vi "Test Acquisition API.vi"() -> ()   [LabVIEW 2019]
doc: "Acquisition API Tester.\n_____\nBased on DQMH Project Template 6.1.0.94."
uses:
  <vilib>/Utility/error.llb/DialogType.ctl
  Acquisition.lvlib
  Settings Editor/Settings Editor.lvlib
panel:
  in  "Command_GndImpedanceData":bool
  in  "Start EOC Acquiring":bool
  in  "Start CNV Acquiring":bool
  in  "IMP data updated":bool
  in  "Start GND Loop acquiring":bool
  in  "Stop IMP acquiring":bool
  in  "Start IMP Acquiring":bool
  in  "Soft Trigger":bool
  in  "Command_GoToIdle":bool
  in  "Command_ImpedanceData":bool
  in  "Command_LiveData":bool
  in  "Command_NoiseData":bool
  in  "Check WiFi AP":bool
  in  "Command_TestData":bool
  in  "Show Diagram on Init":bool
  in  "Settings":bool
  out "error out":errorcluster
  out "Calibrated?":bool
  in  "Calibrate":bool
  out "Waveform Chart":dbl(graph)
  out "Acquiring?":bool
  in  "Stop Acquiring":bool
  out "HW ID":string
  in  "Start Acquiring":bool
  in  "Show Block Diagram":bool
  in  "Stop Module":bool
  in  "Start Module":bool
  in  "Hide Module Panel":bool
  in  "Show Module Panel":bool
  out "Status":string
  out "Module Running?":bool
  # "This VI tests the API for the Module."
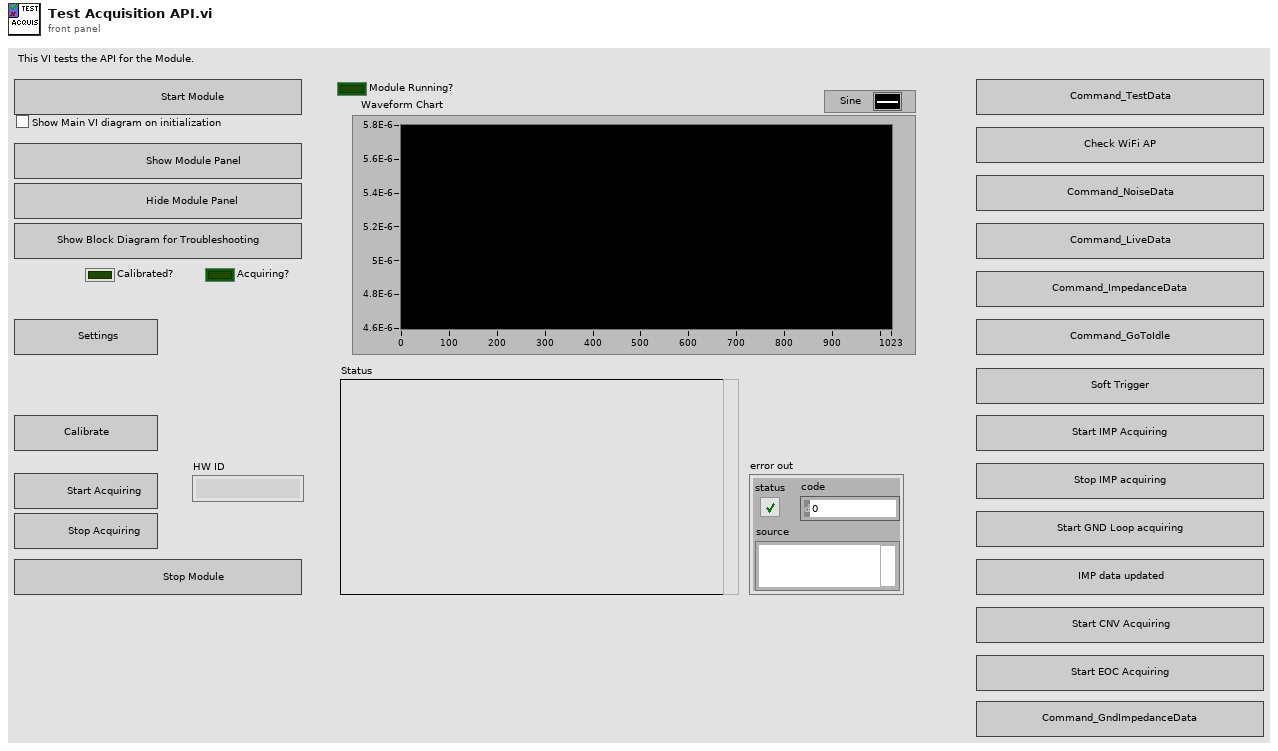
[diagram p1: front panel]
types:
  T1 = typedef "Acquisition.lvlib/Broadcast Events--cluster.ctl" = cluster{"Module Did Init":refnum<user-event>, "Status Updated":refnum<user-event>, "Error Reported":refnum<user-event>, "Module Did Stop":refnum<user-event>, "Update Module Execution Status":refnum<user-event>, "Acquisition Started":refnum<user-event>, "Acquisition Stopped":refnum<user-event>, "Data Updated":refnum<user-event>, "Device Calibrated":refnum<user-event>, "Impedance Data Updated":refnum<user-event>, "CNV Data Updated":refnum<user-event>, "EOC Data Updated":refnum<user-event>}
  T2 = typedef "DialogType.ctl" = u16
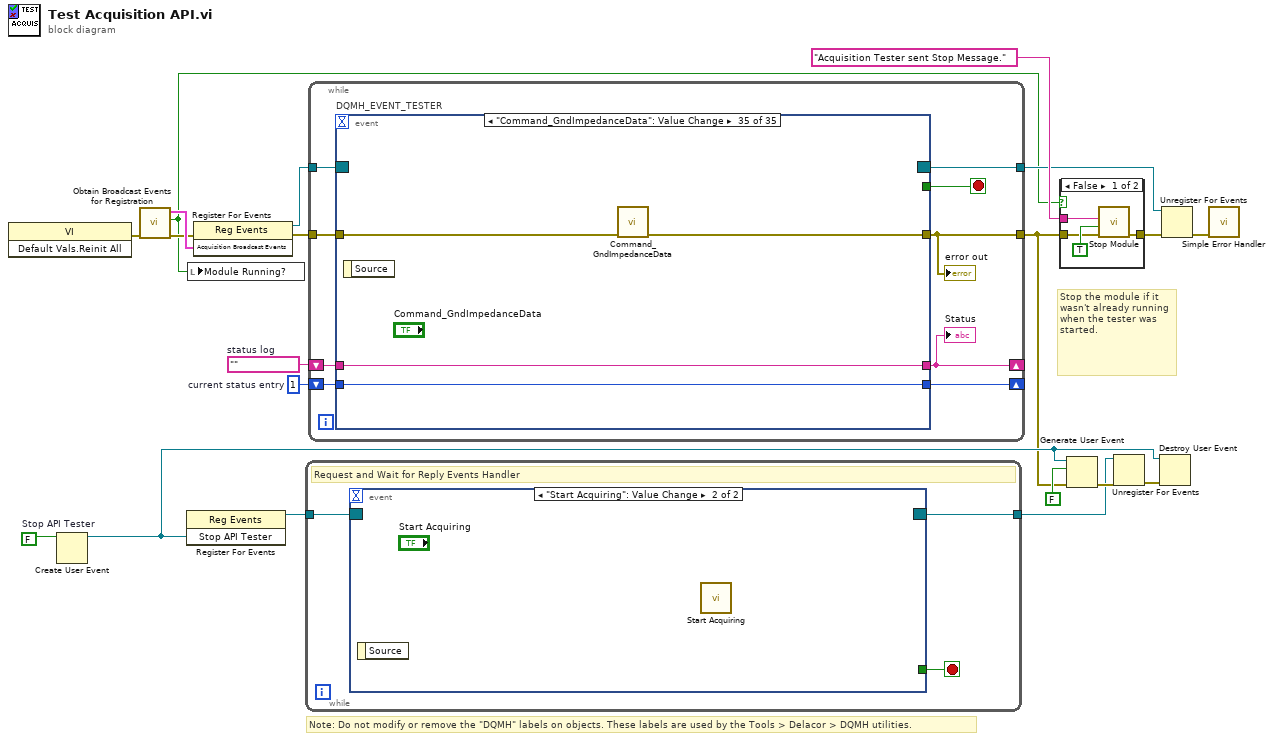
[diagram p0: block diagram]
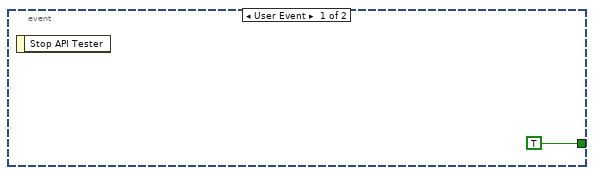
[diagram p2: hidden frame]
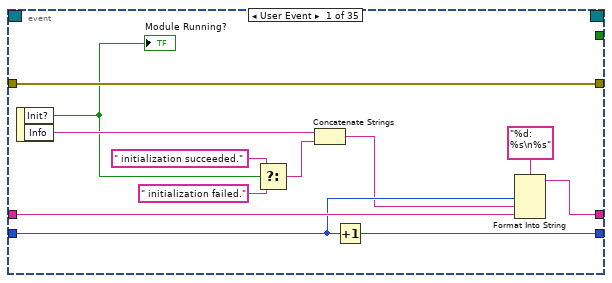
[diagram p3: hidden frame]
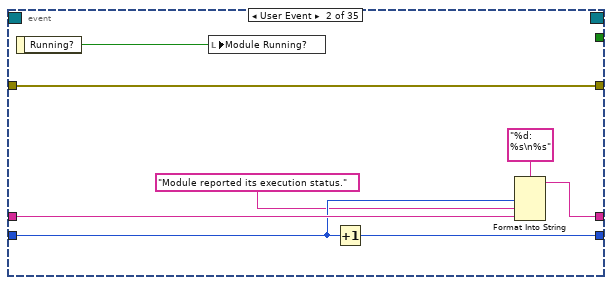
[diagram p4: hidden frame]
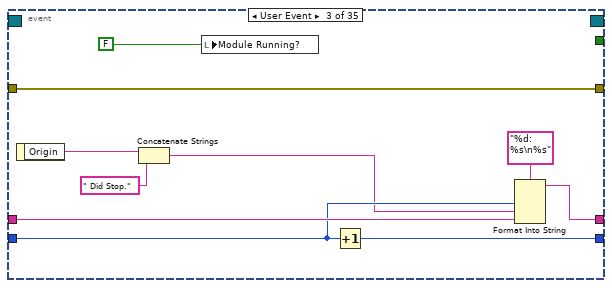
[diagram p5: hidden frame]
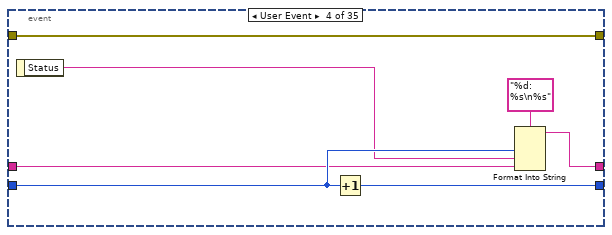
[diagram p6: hidden frame]
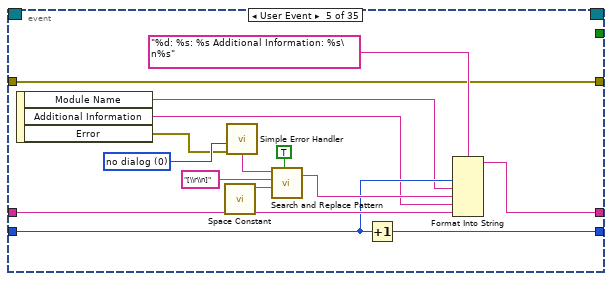
[diagram p7: hidden frame]
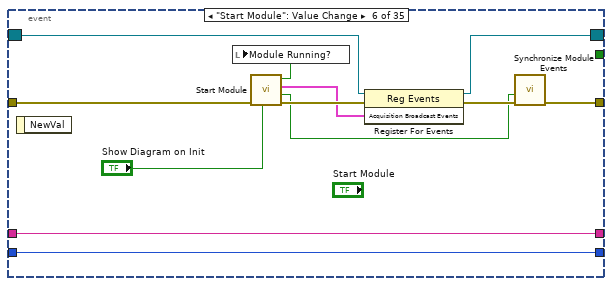
[diagram p8: hidden frame]
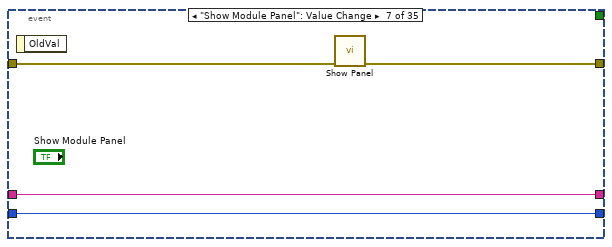
[diagram p9: hidden frame]
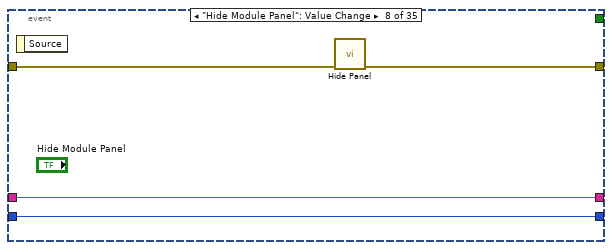
[diagram p10: hidden frame]
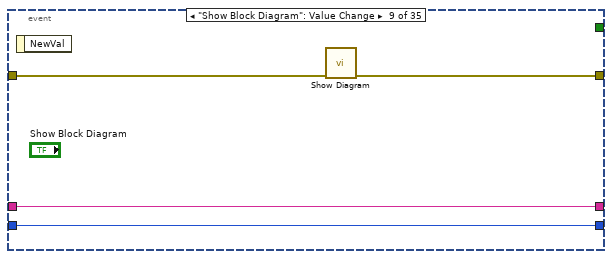
[diagram p11: hidden frame]
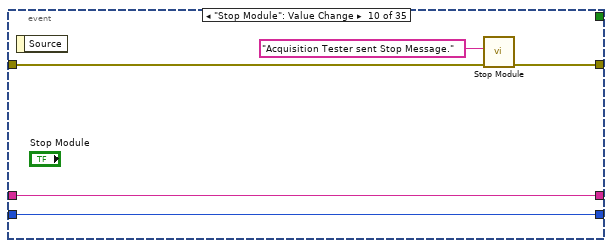
[diagram p12: hidden frame]
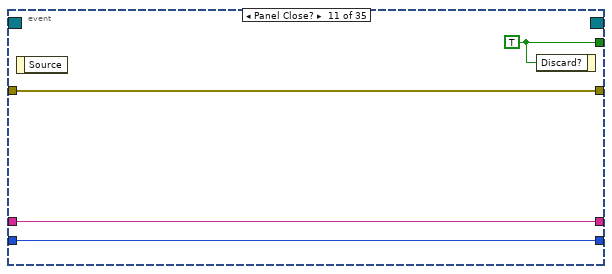
[diagram p13: hidden frame]
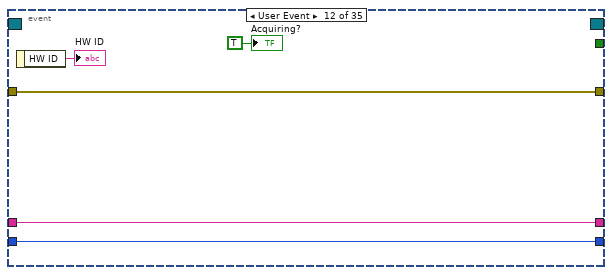
[diagram p14: hidden frame]
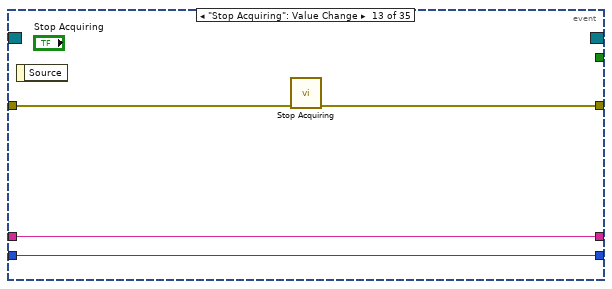
[diagram p15: hidden frame]
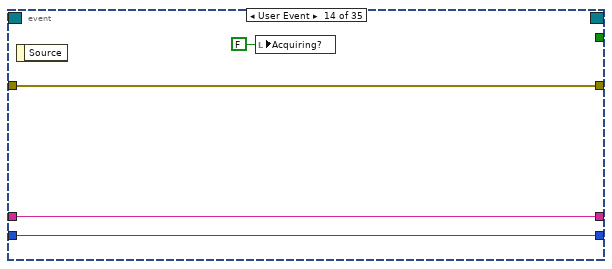
[diagram p16: hidden frame]
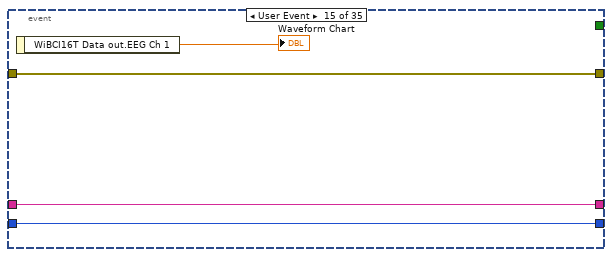
[diagram p17: hidden frame]
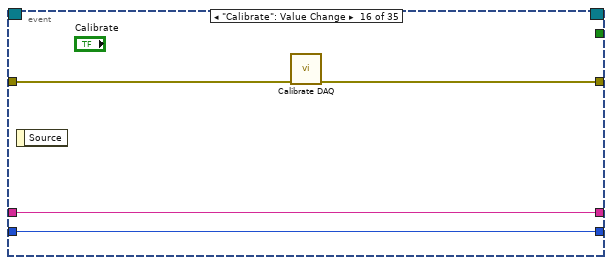
[diagram p18: hidden frame]
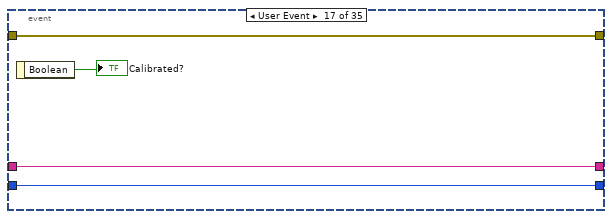
[diagram p19: hidden frame]
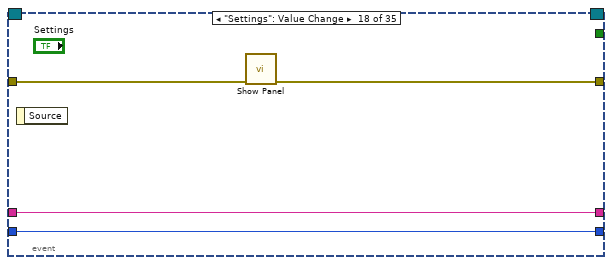
[diagram p20: hidden frame]
diagram:
  w10 = FALSE  # Stop API Tester
  w17 = 1  # current status entry
  w18 = ""  # status log
  # "Stop the module if it wasn't already running when the tester was started."
  # "Note: Do not modify or remove the \"DQMH\" labels on objects. These labels are used by the Tools > Delacor > DQMH utilities."
  n1 = invoke on="Invoke Node" class="VI" method="Default Vals.Reinit All"() -> (error out=w12:errorcluster)  [unwired: 3 in, 2 out]
  n2 = Create User Event(user event datatype=w10) -> (user event=w4:refnum<user-event>)  [unwired: 1 in, 1 out]
  n3 = call "Obtain Broadcast Events for Registration.vi"("error in"=w12) -> ("error out"=w11:errorcluster, "Already running?"=w3:bool, "Acquisition Broadcast Events"=w15:T1)  [unwired: 8 in]
  n4 = register-events(w4) -> (reference out=w9:refnum<event-registration>)  [unwired: 2 in, 1 out]
  n5 = local write "Module Running?"(w3) -> ()
  n6 = register-events(error in=w11, w15) -> (reference out=w14:refnum<event-registration>, error out=w16:errorcluster)  [unwired: 1 in]
  n7 = while {
    tunnel: w9 -> [w23]
    tunnel: [w21] -> w6
    stop <- w22 stop-if-true
    # "Request and Wait for Reply Events Handler"
    n8 = event shown="[1] \"Start Acquiring\": Value Change" {
      selector: w23 -> [_ _]
      dyn-events: [_ _] -> w21
      timeout: _ -> [_ _]
      tunnel: [TRUE _] -> w22
      event User Event {
        n9 = event-data() -> ()  [unwired: 1 in, 1 out]
      }
      event "Start Acquiring": Value Change {
        n10 = event-data() -> ()  [unwired: 1 in, 1 out]
        n11 = call "Start Acquiring.vi"() -> ()  [unwired: 9 in, 3 out]
      }
    }
  }
  n12 = while {
    tunnel: w14 -> [w33]
    tunnel: [w26] -> w2
    shift-right: [w29] -> _
    shift-left: w18 -> [w31]
    shift-right: [w30] -> _
    shift-left: w17 -> [w32]
    tunnel: w16 -> [w28]
    tunnel: [w27] -> w13
    stop <- w25 stop-if-true
    n13 = event "DQMH_EVENT_TESTER" shown="[34] \"Command_GndImpedanceData\": Value Change" {
      selector: w33 -> [_ _ _ _ _ w91 _ _ _ _ _ _ _ _ _ _ _ _ _ _ _ _ _ _ _ _ _ _ _ _ _ _ _ _ _]
      dyn-events: [_ _ _ _ _ w90 _ _ _ _ _ _ _ _ _ _ _ _ _ _ _ _ _ _ _ _ _ _ _ _ _ _ _ _ _] -> w27
      timeout: _ -> [_ _ _ _ _ _ _ _ _ _ _ _ _ _ _ _ _ _ _ _ _ _ _ _ _ _ _ _ _ _ _ _ _ _ _]
      tunnel: [_ _ _ _ _ _ _ _ _ _ w118 _ _ _ _ _ _ _ _ _ _ _ _ _ _ _ _ _ _ _ _ _ _ _ _] -> w25
      tunnel: [w45 w47 w54 w64 w74 w89 w101 w105 w106 w112 w115 w123 w124 w131 w135 w136 w143 w144 w148 w152 w156 w160 w164 w168 w173 w177 w181 w185 w189 w199 w208 w209 w213 w225 w226] -> w26
      tunnel: w32 -> [w42 w51 w61 w67 w77 w94 w99 w103 w107 w113 w116 w121 w125 w129 w133 w137 w141 w146 w149 w153 w157 w161 w165 w169 w174 w178 w182 w186 w190 w196 w205 w210 w214 w222 w227]
      tunnel: w31 -> [w43 w52 w62 w66 w78 w95 w100 w104 w108 w114 w117 w122 w126 w130 w134 w138 w142 w147 w150 w154 w158 w162 w166 w170 w175 w179 w183 w187 w191 w198 w207 w211 w215 w224 w228]
      tunnel: [w40 w49 w59 w68 w75 w95 w100 w104 w108 w114 w117 w122 w126 w130 w134 w138 w142 w147 w150 w154 w158 w162 w166 w170 w175 w179 w183 w187 w191 w197 w206 w211 w215 w223 w228] -> w29
      tunnel: [w41 w50 w60 w70 w76 w94 w99 w103 w107 w113 w116 w121 w125 w129 w133 w137 w141 w146 w149 w153 w157 w161 w165 w169 w174 w178 w182 w186 w190 w195 w204 w210 w214 w221 w227] -> w30
      tunnel: w28 -> [w45 w47 w54 w64 w74 w88 w98 w102 w109 w110 w115 w123 w127 w131 w135 w139 w143 w145 w151 w155 w159 w163 w167 w171 w176 w180 w184 w188 w192 w199 w208 w212 w216 w225 w229]
      event User Event {
        n14 = event-data() -> ("Init?"=w37:bool, "Info"=w39:string)  [unwired: 1 in]
        "Module Running?" <- w37
        n15 = Select(t=" initialization succeeded.", s=w37, f=" initialization failed.") -> (s? t:f=w34:string)
        n16 = Concatenate Strings(w39, w34) -> (w38:string)
        n17 = Increment(x=w42) -> (x+1=w41:i32)
        n18 = Format Into String(format string="%d: %s\n%s", w42, w38, w43) -> (resulting string=w40:string)  [unwired: 2 in, 1 out]
      }
      event User Event {
        n19 = event-data() -> ("Running?"=w46:bool)  [unwired: 1 in]
        n20 = local write "Module Running?"(w46) -> ()
        n21 = Increment(x=w51) -> (x+1=w50:i32)
        n22 = Format Into String(format string="%d: %s\n%s", w51, "Module reported its execution status.", w52) -> (resulting string=w49:string)  [unwired: 2 in, 1 out]
      }
      event User Event {
        n23 = event-data() -> ("Origin"=w58:string)  [unwired: 1 in]
        n24 = Concatenate Strings(w58, " Did Stop.") -> (w57:string)
        n25 = local write "Module Running?"(FALSE ("Module Did Init?")) -> ()
        n26 = Increment(x=w61) -> (x+1=w60:i32)
        n27 = Format Into String(format string="%d: %s\n%s", w61, w57, w62) -> (resulting string=w59:string)  [unwired: 2 in, 1 out]
      }
      event User Event {
        n28 = event-data() -> ("Status"=w65:string)  [unwired: 1 in]
        n29 = Increment(x=w67) -> (x+1=w70:i32)
        n30 = Format Into String(format string="%d: %s\n%s", w67, w65, w66) -> (resulting string=w68:string)  [unwired: 2 in, 1 out]
      }
      event User Event {
        w79 = T2 0 items=["no dialog", "OK message", "continue or stop message", "OK message + warnings", "continue/stop + warnings"] ("type of dialog (OK msg:1)")
        n31 = event-data() -> ("Module Name"=w73:string, "Additional Information"=w72:string, "Error"=w71:errorcluster)  [unwired: 1 in]
        n32 = call <vilib>:"Space Constant.vi"() -> ("String"=w83:string)
        n33 = call <vilib>:"Simple Error Handler.vi"("type of dialog (OK msg:1)"=w79, "error in (no error)"=w71) -> ("message"=w80:string)  [unwired: 3 in, 4 out]
        n34 = call <vilib>:"Search and Replace Pattern.vi"("string"=w80, "regular expression (\"\")"="[\\r\\n]" ("regular expression (\"\")"), "replace string (\"\")"=w83, "replace all? (F)"=TRUE ("replace all CR/LF with spaces")) -> ("result string"=w81:string)  [unwired: 1 in, 1 out]
        n35 = Increment(x=w77) -> (x+1=w76:i32)
        n36 = Format Into String(format string="%d: %s: %s Additional Information: %s\n%s", w77, w73, w81, w72, w78) -> (resulting string=w75:string)  [unwired: 2 in, 1 out]
      }
      event "Start Module": Value Change {
        n37 = event-data() -> ()  [unwired: 1 in, 1 out]
        n38 = call "Start Module.vi"("Show Main VI Diagram on Init (F)"="Show Diagram on Init", "error in"=w88) -> ("error out"=w96:errorcluster, "Wait for Event Sync?"=w93:bool, "Acquisition Broadcast Events"=w92:T1, "Module Was Already Running?"=w87:bool)  [unwired: 6 in]
        n39 = local write "Module Running?"(w87) -> ()
        n40 = register-events(reference=w91, error in=w96, w92) -> (reference out=w90:refnum<event-registration>, error out=w97:errorcluster)
        n41 = call "Synchronize Module Events.vi"("error in (no error)"=w97, "Wait for Event Sync?"=w93) -> ("error out"=w89:errorcluster)  [unwired: 9 in]
      }
      event "Show Module Panel": Value Change {
        n42 = event-data() -> ()  [unwired: 1 in, 1 out]
        n43 = call "Show Panel.vi"("error in (no error)"=w98) -> ("error out"=w101:errorcluster)  [unwired: 10 in]
      }
      event "Hide Module Panel": Value Change {
        n44 = event-data() -> ()  [unwired: 1 in, 1 out]
        n45 = call "Hide Panel.vi"("error in (no error)"=w102) -> ("error out"=w105:errorcluster)  [unwired: 10 in]
      }
      event "Show Block Diagram": Value Change {
        n46 = event-data() -> ()  [unwired: 1 in, 1 out]
        n47 = call "Show Diagram.vi"("error in (no error)"=w109) -> ("error out"=w106:errorcluster)  [unwired: 10 in]
      }
      event "Stop Module": Value Change {
        n48 = event-data() -> ()  [unwired: 1 in, 1 out]
        n49 = call "Stop Module.vi"("error in"=w110, "Origin"="Acquisition Tester sent Stop Message.") -> ("error out"=w112:errorcluster)  [unwired: 9 in]
      }
      event Panel Close? {
        w118 = TRUE ("Discard?")
        n50 = event-data() -> ()  [unwired: 1 in, 1 out]
        n51 = event-data ("Event Filter Node")("Discard?"=w118) -> ()  [unwired: 1 in, 1 out]
      }
      event User Event {
        n52 = event-data() -> ("HW ID"=→"HW ID":string)  [unwired: 1 in]
        "Acquiring?" <- TRUE ("Acquiring?")
      }
      event "Stop Acquiring": Value Change {
        n53 = event-data() -> ()  [unwired: 1 in, 1 out]
        n54 = call "Stop Acquiring.vi"("error in (no error)"=w127) -> ("error out"=w124:errorcluster)  [unwired: 10 in]
      }
      event User Event {
        n55 = event-data() -> ()  [unwired: 1 in, 1 out]
        n56 = local write "Acquiring?"(FALSE ("Acquiring?")) -> ()
      }
      event User Event {
        n57 = event-data() -> ("WiBCI16T Data out.EEG Ch 1"=→"Waveform Chart":dbl)  [unwired: 1 in]
      }
      event "Calibrate": Value Change {
        n58 = event-data() -> ()  [unwired: 1 in, 1 out]
        n59 = call "Calibrate DAQ.vi"("error in (no error)"=w139) -> ("error out"=w136:errorcluster)  [unwired: 10 in]
      }
      event User Event {
        n60 = event-data() -> ("Boolean"=→"Calibrated?":bool)  [unwired: 1 in]
      }
      event "Settings": Value Change {
        n61 = event-data() -> ()  [unwired: 1 in, 1 out]
        n62 = call "Show Panel.vi"("error in (no error)"=w145) -> ("error out"=w144:errorcluster)  [unwired: 10 in]
      }
      event "Command_TestData": Value Change {
        # "#CodeNeeded\n1. Position the new \"Command_TestData\" button appropriately on the front panel.\n2. Delete or edit this label when done."
        n63 = event-data() -> ()  [unwired: 1 in, 1 out]
        n64 = call "Command_TestData.vi"("error in"=w151) -> ("error out"=w148:errorcluster)  [unwired: 10 in]
      }
      event "Check WiFi AP": Value Change {
        # "#CodeNeeded\n1. Position the new \"Check WiFi AP\" button appropriately on the front panel.\n2. Delete or edit this label when done."
        n65 = event-data() -> ()  [unwired: 1 in, 1 out]
        n66 = call "Check WiFi AP.vi"("error in"=w155) -> ("error out"=w152:errorcluster)  [unwired: 10 in]
      }
      event "Command_NoiseData": Value Change {
        # "#CodeNeeded\n1. Position the new \"Command_NoiseData\" button appropriately on the front panel.\n2. Delete or edit this label when done."
        n67 = event-data() -> ()  [unwired: 1 in, 1 out]
        n68 = call "Command_NoiseData.vi"("error in"=w159) -> ("error out"=w156:errorcluster)  [unwired: 10 in]
      }
      event "Command_LiveData": Value Change {
        # "#CodeNeeded\n1. Position the new \"Command_LiveData\" button appropriately on the front panel.\n2. Delete or edit this label when done."
        n69 = event-data() -> ()  [unwired: 1 in, 1 out]
        n70 = call "Command_LiveData.vi"("error in"=w163) -> ("error out"=w160:errorcluster)  [unwired: 10 in]
      }
      event "Command_ImpedanceData": Value Change {
        # "#CodeNeeded\n1. Position the new \"Command_ImpedanceData\" button appropriately on the front panel.\n2. Delete or edit this label when done."
        n71 = event-data() -> ()  [unwired: 1 in, 1 out]
        n72 = call "Command_ImpedanceData.vi"("error in"=w167) -> ("error out"=w164:errorcluster)  [unwired: 10 in]
      }
      event "Command_GoToIdle": Value Change {
        # "#CodeNeeded\n1. Position the new \"Command_GoToIdle\" button appropriately on the front panel.\n2. Delete or edit this label when done."
        n73 = event-data() -> ()  [unwired: 1 in, 1 out]
        n74 = call "Command_GoToIdle.vi"("error in"=w171) -> ("error out"=w168:errorcluster)  [unwired: 10 in]
      }
      event "Soft Trigger": Value Change {
        n75 = event-data() -> ()  [unwired: 1 in, 1 out]
        n76 = call "Soft Trigger.vi"("error in"=w176, "Value"=i8 100) -> ("error out"=w173:errorcluster)  [unwired: 9 in]
      }
      event "Start IMP Acquiring": Value Change {
        # "#CodeNeeded\n1. Position the new \"Start IMP Acquiring\" button appropriately on the front panel.\n2. Delete or edit this label when done."
        n77 = event-data() -> ()  [unwired: 1 in, 1 out]
        n78 = call "Start IMP Acquiring.vi"("error in"=w180) -> ("error out"=w177:errorcluster)  [unwired: 10 in]
      }
      event "Stop IMP acquiring": Value Change {
        # "#CodeNeeded\n1. Position the new \"Stop IMP acquiring\" button appropriately on the front panel.\n2. Delete or edit this label when done."
        n79 = event-data() -> ()  [unwired: 1 in, 1 out]
        n80 = call "Stop IMP acquiring.vi"("error in"=w184) -> ("error out"=w181:errorcluster)  [unwired: 10 in]
      }
      event "Start GND Loop acquiring": Value Change {
        # "#CodeNeeded\n1. Position the new \"Start GND Loop acquiring\" button appropriately on the front panel.\n2. Delete or edit this label when done."
        n81 = event-data() -> ()  [unwired: 1 in, 1 out]
        n82 = call "Start GND Loop acquiring.vi"("error in"=w188) -> ("error out"=w185:errorcluster)  [unwired: 10 in]
      }
      event "IMP data updated": Value Change {
        # "#CodeNeeded\n1. Position the new \"IMP data updated\" button appropriately on the front panel.\n2. Delete or edit this label when done."
        n83 = event-data() -> ()  [unwired: 1 in, 1 out]
        n84 = call "IMP data updated.vi"("error in"=w192) -> ("error out"=w189:errorcluster)  [unwired: 8 in, 2 out]
      }
      event User Event {
        n85 = event-data() -> ()  [unwired: 1 in, 5 out]
        n86 = Increment(x=w196) -> (x+1=w195:i32)
        n87 = Format Into String(format string="%d: %s\n%s", w196, "Impedance Data Updated" ("input 2"), w198) -> (resulting string=w197:string)  [unwired: 2 in, 1 out]
      }
      event User Event {
        # "#CodeNeeded\n1. Process the event data sent by the \"CNV Data Updated\" broadcast event.\n2. Delete or edit this label when done."
        n88 = event-data() -> ()  [unwired: 1 in, 6 out]
        n89 = Format Into String(format string="Response Received - %s", "CNV Data Updated" ("input 1")) -> (resulting string=w201:string)  [unwired: 2 in, 1 out]
        n90 = Increment(x=w205) -> (x+1=w204:i32)
        n91 = Format Into String(format string="%d: %s\n%s", w205, w201, w207) -> (resulting string=w206:string)  [unwired: 2 in, 1 out]
      }
      event "Start CNV Acquiring": Value Change {
        n92 = event-data() -> ()  [unwired: 1 in, 1 out]
        n93 = call "Start CNV Acquiring.vi"("error in"=w212) -> ("error out"=w209:errorcluster)  [unwired: 10 in]
      }
      event "Start EOC Acquiring": Value Change {
        n94 = event-data() -> ()  [unwired: 1 in, 1 out]
        n95 = call "Start EOC Acquiring.vi"("error in"=w216) -> ("error out"=w213:errorcluster)  [unwired: 10 in]
      }
      event User Event {
        n96 = event-data() -> ()  [unwired: 1 in, 5 out]
        n97 = Format Into String(format string="Response Received - %s", "EOC Data Updated" ("input 1")) -> (resulting string=w218:string)  [unwired: 2 in, 1 out]
        n98 = Increment(x=w222) -> (x+1=w221:i32)
        n99 = Format Into String(format string="%d: %s\n%s", w222, w218, w224) -> (resulting string=w223:string)  [unwired: 2 in, 1 out]
      }
      event "Command_GndImpedanceData": Value Change {
        n100 = event-data() -> ()  [unwired: 1 in, 1 out]
        n101 = call "Command_GndImpedanceData.vi"("error in"=w229) -> ("error out"=w226:errorcluster)  [unwired: 10 in]
      }
    }
    "Status" <- w29
    "error out" <- w26
  }
  n102 = case shown="False" w3 {
    tunnel: [w233 w234] -> w20
    tunnel: "Acquisition Tester sent Stop Message." ("Origin") -> [w232 _]
    tunnel: w2 -> [w230 w234]
    frame False {
      n103 = call "Stop Module.vi"("error in"=w230, "Wait for Module to Stop? (F)"=TRUE ("Wait for Module to stop?"), "Origin"=w232) -> ("error out"=w233:errorcluster)  [unwired: 8 in]
    }
    frame True {
    }
  }
  n104 = Generate User Event(user event=w4, event data cluster=FALSE ("Stop API Tester"), error in=w2) -> (error out=w7:errorcluster)  [unwired: 1 in, 1 out]
  n105 = Unregister For Events(event registration refnum=w6, error in=w7) -> (error out=w5:errorcluster)
  n106 = Destroy User Event(user event=w4, error in=w5) -> ()  [unwired: 1 out]
  n107 = Unregister For Events(event registration refnum=w13, error in=w20) -> (error out=w1:errorcluster)
  n108 = call <vilib>:"Simple Error Handler.vi"("error in (no error)"=w1) -> ()  [unwired: 4 in, 5 out]
